vi "Parse Raw Frame.vi"(10 "Data":u8[](array[numeric]) format="%.0x", 11 "HeaderInfo":T2={"InterFrameGap"=0, "PacketGroupWaitTime"=10000, "PayloadBufferMode"=0, "PayloadGenerationMode"=0, "PreambleCount"=7, "Skew"=0, "NetSelect"=4, "FrameStartMode"=1, "PhysErrorInjection"=0, "SequenceNumberInit"=65535, "SequenceNumberOffset"=65535} {"NetSelect" items=["FDX_TX_FRAME_DLY_A"=0, "FDX_TX_FRAME_DLY_B"=1, "FDX_TX_FRAME_BOTH "=3, "FDX_TX_FRAME_ONLY_A"=4, "FDX_TX_FRAME_ONLY_B "=5]; "FrameStartMode" items=["FDX_TX_FRAME_START_IFG", "FDX_TX_FRAME_START_PGWT", "FDX_TX_FRAME_START_TRG"]; "PhysErrorInjection" items=["FDX_TX_FRAME_ERR_OFF"=0, "FDX_TX_FRAME_ERR_CRC"=1, "FDX_TX_FRAME_ERR_ALI"=2, "FDX_TX_FRAME_ERR_PRE"=4, "FDX_TX_FRAME_ERR_PHY"=8]; "SequenceNumberInit" items=["FDX_TX_FRAME_SEQ_INIT_AUTO"=65535]; "SequenceNumberOffset" items=["FDX_TX_FRAME_SEQ_OFFS_AUTO "=65535]; "PayloadGenerationMode" items=["FDX_TX_FRAME_PGM_USER"=0, "FDX_TX_FRAME_PGM_IP_PART"=1, "FDX_TX_FRAME_PGM_IP_FULL"=2, "FDX_TX_FRAME_PGM_IP_PART_TT"=10, "FDX_TX_FRAME_PGM_IP_FULL_TT"=20]; "PayloadBufferMode" items=["FDX_TX_FRAME_PBM_STD", "FDX_TX_FRAME_PBM_MAC", "FDX_TX_FRAME_PBM_UDP"]}) -> (0 "UDPsrcPort":u16=1, 1 "UDPdstPort":u16=1, 2 "VL Id":u16=60, 3 "Payload":u8[](array[numeric]), 5 "Frame Configuration":T1={"domainID"=1, "sideID"=1, "locationID"=1, "interfaceID"=1, "partitionID"=1} {"interfaceID" format="%.0b"})   [LabVIEW 2020]
uses:
  <instrlib>/AIM GmbH/_AIM 664/_controls/queue_header_generic.ctl
  <instrlib>/AIM GmbH/_AIM 664/_controls/queue_data_full.ctl
  <instrlib>/AIM GmbH/_AIM 664/helpers/EthFrameManagement/EthFrameManagement.lvlib
  <instrlib>/AIM GmbH/_AIM 664/AIM664LV.lvlib
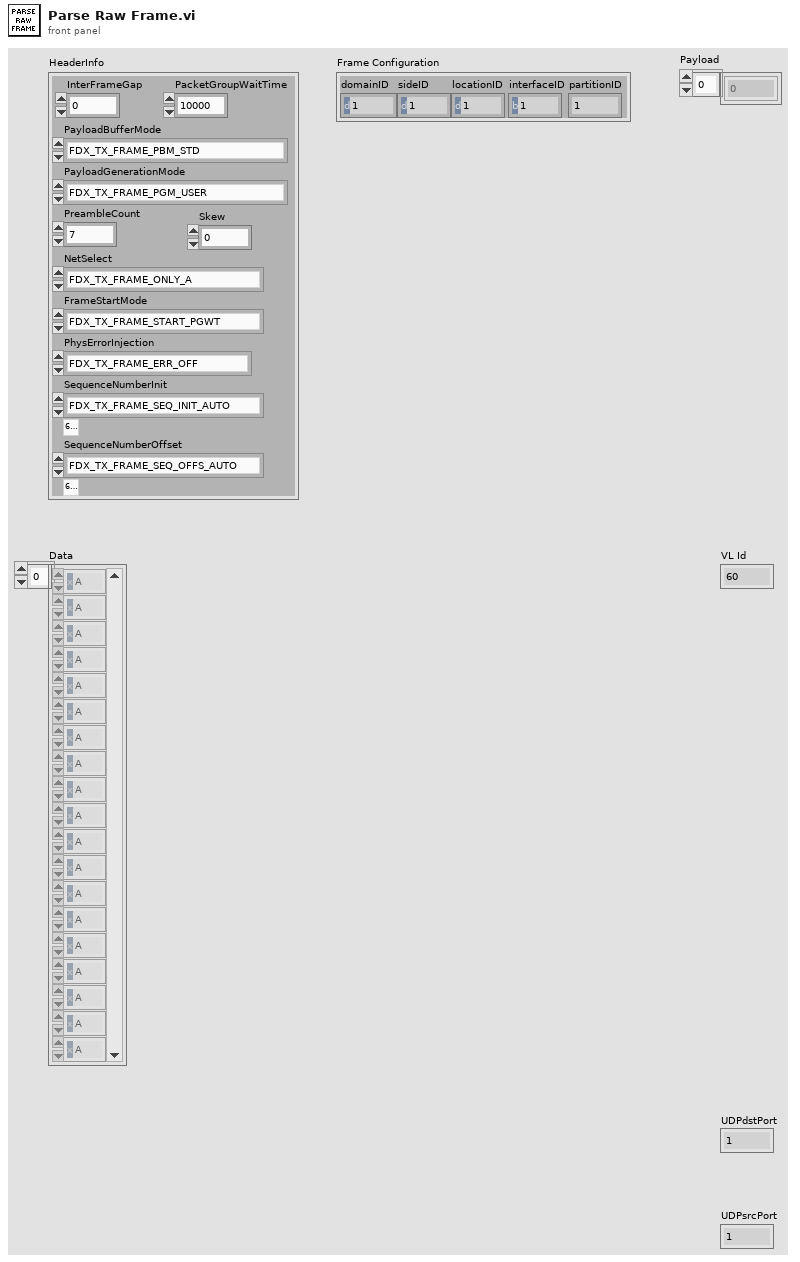
[diagram p1: front panel]
types:
  T1 = typedef "AIM664LV.lvlib/queue_data_full.ctl" = cluster{"domainID":u8, "sideID":u8, "locationID":u8, "interfaceID":u8, "partitionID":u8}
  T2 = typedef "AIM664LV.lvlib/queue_header_generic.ctl" = cluster{"InterFrameGap":u32, "PacketGroupWaitTime":u32, "PayloadBufferMode":u8, "PayloadGenerationMode":u8, "PreambleCount":u8, "Skew":u32, "NetSelect":u8, "FrameStartMode":u8, "PhysErrorInjection":u32, "SequenceNumberInit":u16, "SequenceNumberOffset":u16}
  T3 = typedef "EthFrameManagement.lvlib/ehternetFrame_type.ctl" = cluster{"Dest MAC":u8[], "Src MAC":u8[], "EtherType":u16}
  T4 = typedef "EthFrameManagement.lvlib/UDPFrame_type.ctl" = cluster{"Source Port":u16, "Dest Port":u16, "Lenght":u16, "Checksum":u16}
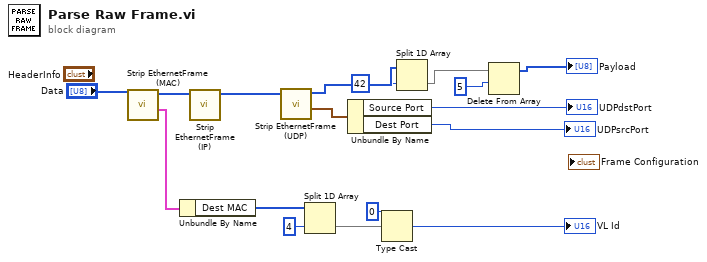
[diagram p0: block diagram]
diagram:
  n1 = call <instrlib>:"Strip EthernetFrame (MAC).vi"("Ethernet Frame In"="Data") -> ("Ethernet header"=w14:T3, "Ethernet Frame Out"=w16:u8[])  [unwired: 7 in, 2 out]
  n2 = Unbundle By Name(w14) -> ("Dest MAC"=w10:u8[])
  n3 = call <instrlib>:"Strip EthernetFrame (IP).vi"("Frame In"=w16) -> ("Frame Out"=w15:u8[])  [unwired: 7 in, 3 out]
  n4 = call <instrlib>:"Strip EthernetFrame (UDP).vi"("Ethernet Frame In"=w15) -> ("UDP header"=w13:T4, "Ethernet Frame Out"=w5:u8[])  [unwired: 7 in, 2 out]
  n5 = Split 1D Array(array=w10, index=4) -> (second subarray=w7:u8[])  [unwired: 1 out]
  n6 = Unbundle By Name(w13) -> ("Source Port"=→"UDPdstPort":u16, "Dest Port"=→"UDPsrcPort":u16)
  n7 = Type Cast(type=u16 0 ("VL Id 2"), x=w7) -> (*(type *) &x=→"VL Id":u16)
  n8 = Split 1D Array(array=w5, index=42) -> (second subarray=w2:u8[])  [unwired: 1 out]
  n9 = Delete From Array(array=w2, length=5 ("index")) -> (array with subset deleted=→"Payload":u8[])  [unwired: 1 in, 1 out]
